vi "GBF Face avant.vi"() -> ()   [LabVIEW 2024]
uses:
  <vilib>/measure/NI_MABase.lvlib
panel:
  in  "reset signal":bool caption="réinitialisation du signal"
  out "Fréquence":dbl
  in  "N° octave":u8(knob) max=9 step=1 scale=0.0..9.0
  in  "Sib":bool
  in  "Sol#":bool
  in  "Fa#":bool
  in  "Mib":bool
  in  "Do#":bool
  in  "SI":bool
  in  "LA":bool
  in  "SOL":bool
  in  "FA":bool
  in  "MI":bool
  in  "RE":bool
  in  "DO":bool
  in  "signal type":T1(ring) caption="type de signal"
  in  "Atténuation":bool
  in  "sampling info":cluster{"Fs":dbl, "#s":dbl}={"Fs"=100000.0, "#s"=100000.0} caption="Echantillonnage" {"Fs" format="%.2p"}
  in  "Bouton Stop":bool
  out "Signal":waveform(dbl)(graph)={"t0"=timestamp(56 s since 1904-01-01), "dt"=1e-05, "Y"=array[100000 elements]}
  in  "Rapport cyclique (%)":dbl(slide) min=0.0 max=100.0 step=5.0 scale=0.0..100.0
  in  "Amplitude":dbl(knob) min=0.0 max=1.0 step=0.01 scale=0.0..1.0
  # "GENERATEUR 1 OCTAVE"
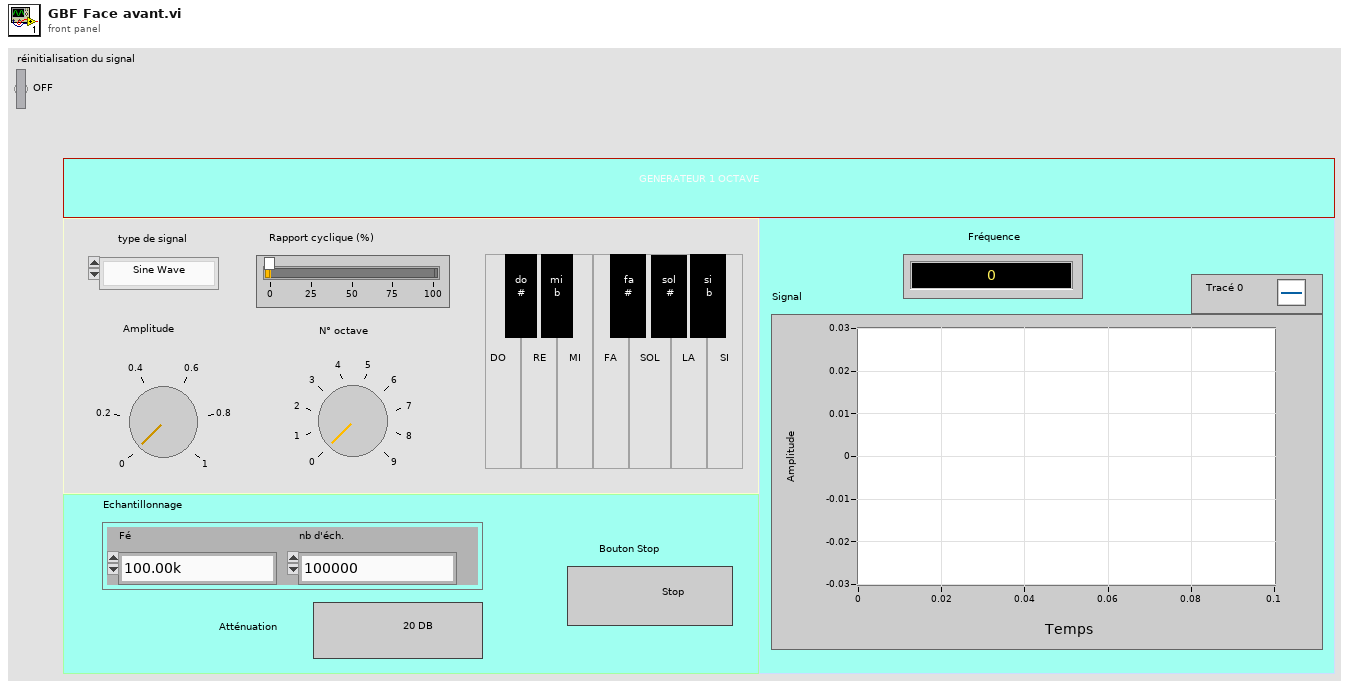
[diagram p1: front panel]
types:
  T1 = enum16{"Sine Wave", "Triangle Wave", "Square Wave", "Sawtooth Wave"}
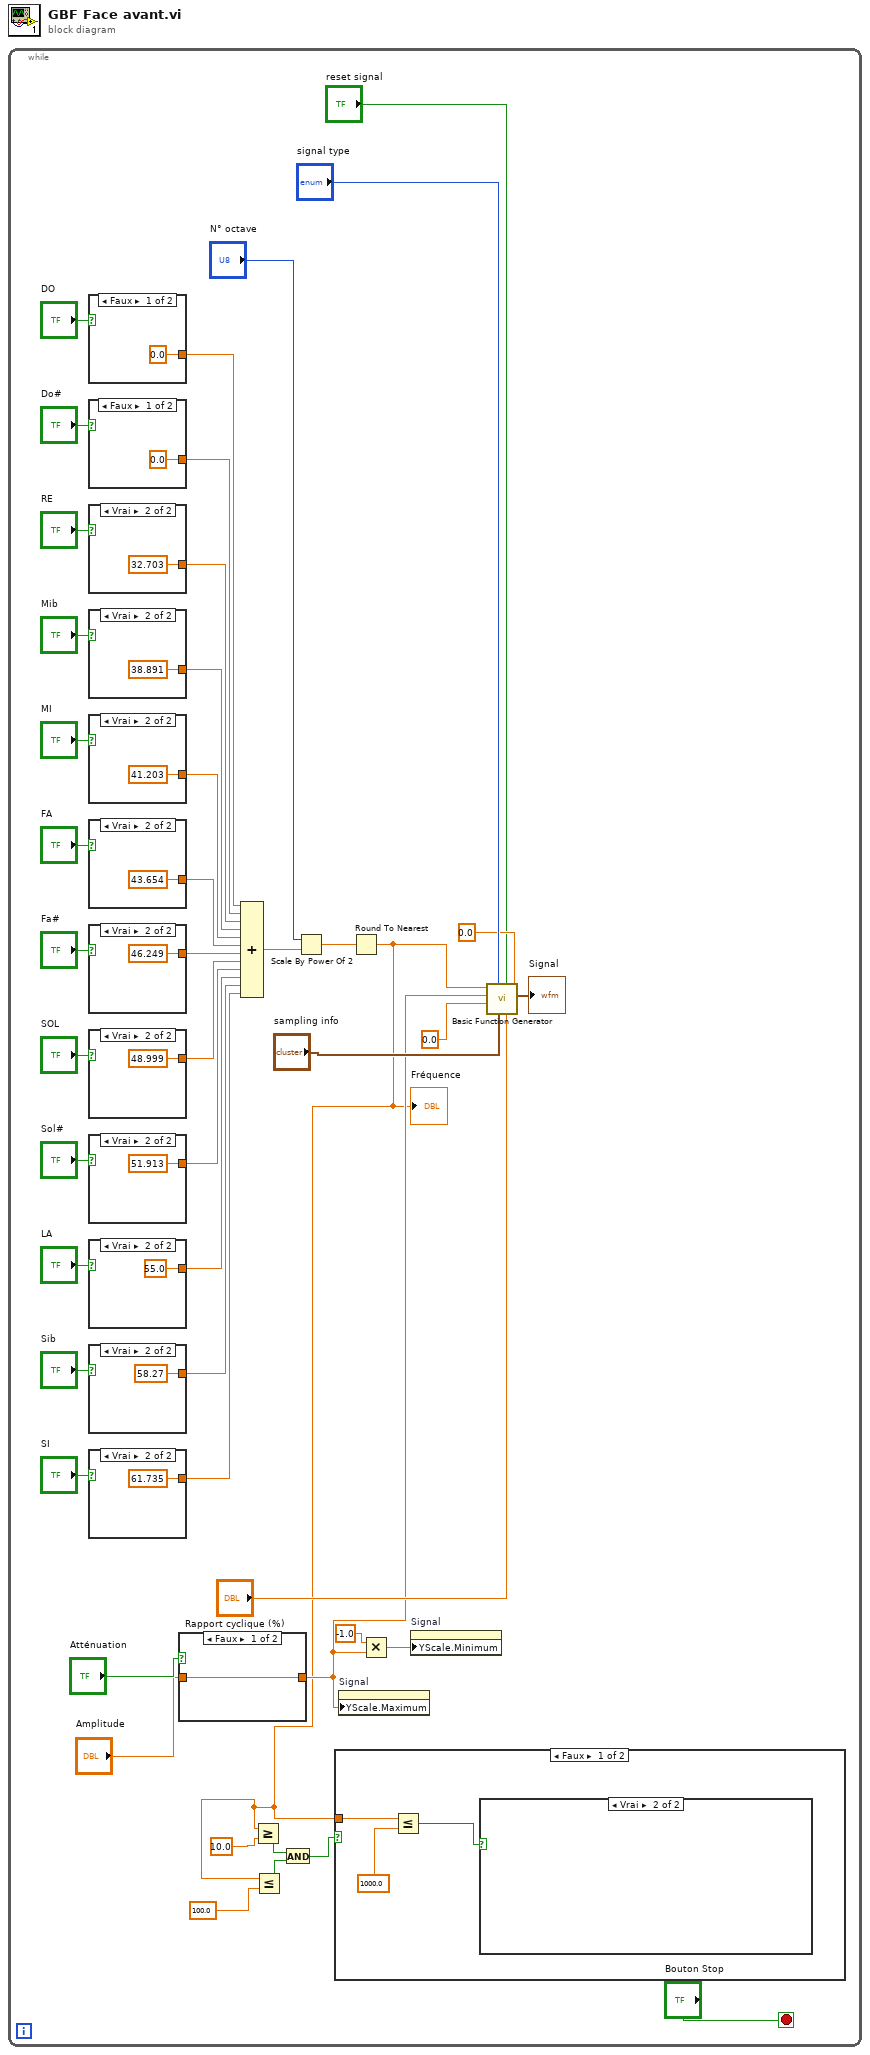
[diagram p0: block diagram]
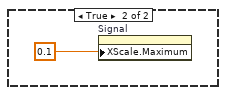
[diagram p3: hidden frame]
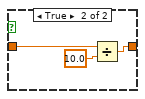
[diagram p4: hidden frame]
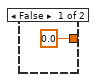
[diagram p5: hidden frame]
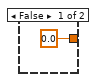
[diagram p6: hidden frame]
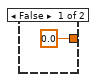
[diagram p7: hidden frame]
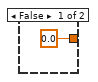
[diagram p8: hidden frame]
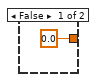
[diagram p9: hidden frame]
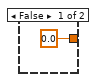
[diagram p10: hidden frame]
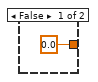
[diagram p11: hidden frame]
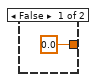
[diagram p12: hidden frame]
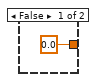
[diagram p13: hidden frame]
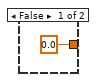
[diagram p14: hidden frame]
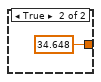
[diagram p15: hidden frame]
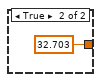
[diagram p16: hidden frame]
diagram:
  n1 = while {
    stop <- "Bouton Stop" stop-if-true
    n2 = case shown="Faux" "DO" {
      tunnel: [0.0 32.703] -> w28
      frame False {
      }
      frame True {
      }
    }
    n3 = case shown="Faux" "Do#" {
      tunnel: [0.0 34.648] -> w27
      frame False {
      }
      frame True {
      }
    }
    n4 = case shown="Vrai" "RE" {
      tunnel: [0.0 32.703] -> w26
      frame False {
      }
      frame True {
      }
    }
    n5 = case shown="Vrai" "Mib" {
      tunnel: [0.0 38.891] -> w25
      frame False {
      }
      frame True {
      }
    }
    n6 = case shown="Vrai" "MI" {
      tunnel: [0.0 41.203] -> w24
      frame False {
      }
      frame True {
      }
    }
    n7 = case shown="Vrai" "FA" {
      tunnel: [0.0 43.654] -> w23
      frame False {
      }
      frame True {
      }
    }
    n8 = case shown="Vrai" "Fa#" {
      tunnel: [0.0 46.249] -> w22
      frame False {
      }
      frame True {
      }
    }
    n9 = case shown="Vrai" "SOL" {
      tunnel: [0.0 48.999] -> w21
      frame False {
      }
      frame True {
      }
    }
    n10 = case shown="Vrai" "Sol#" {
      tunnel: [0.0 51.913] -> w20
      frame False {
      }
      frame True {
      }
    }
    n11 = case shown="Vrai" "LA" {
      tunnel: [0.0 55.0] -> w19
      frame False {
      }
      frame True {
      }
    }
    n12 = case shown="Vrai" "Sib" {
      tunnel: [0.0 58.27] -> w18
      frame False {
      }
      frame True {
      }
    }
    n13 = case shown="Vrai" "SI" {
      tunnel: [0.0 61.735] -> w17
      frame False {
      }
      frame True {
      }
    }
    n14 = case shown="Faux" "Atténuation" {
      tunnel: [w51 w54] -> w8
      tunnel: "Amplitude" -> [w51 w53]
      frame False {
      }
      frame True {
        n15 = Divide(x=w53, y=10.0) -> (x/y=w54:dbl)
      }
    }
    n16 = Compound Arithmetic op=ADD(w28, w27, w26, w25, w24, w23, w22, w21, w20, w19, w18, w17) -> (w16:dbl)
    n17 = Scale By Power Of 2(n="N° octave", x=w16) -> (x*2^n=w10:dbl)
    n18 = property on="Signal" class="GraphWF (strict)"("YScale.Maximum"=w8) -> ()  [unwired: 2 in, 2 out]
    n19 = Round To Nearest(number=w10) -> (nearest integer value=w1:dbl)
    "Fréquence" <- w1
    n20 = Greater Or Equal?(x=w1, y=10.0) -> (x >= y?=w4:bool)
    n21 = Less Or Equal?(x=w1, y=100.0) -> (x <= y?=w3:bool)
    n22 = And(x=w4, y=w3) -> (x .and. y?=w2:bool)
    n23 = case shown="Faux" w2 {
      tunnel: w1 -> [w48 _]
      frame False {
        n24 = Less Or Equal?(x=w48, y=1000.0) -> (x <= y?=w49:bool)
        n25 = case shown="Vrai" w49 {
          frame False {
          }
          frame True {
          }
        }
      }
      frame True {
        n26 = property on="Signal" class="GraphWF (strict)"("XScale.Maximum"=0.1) -> ()  [unwired: 2 in, 2 out]
      }
    }
    n27 = Multiply(x=-1.0, y=w8) -> (x*y=w7:dbl)
    n28 = property on="Signal" class="GraphWF (strict)"("YScale.Minimum"=w7) -> ()  [unwired: 2 in, 2 out]
    n29 = call <vilib>:"Basic Function Generator.vi"("offset"=0.0, "square wave duty cycle (%)"="Rapport cyclique (%)", "reset signal"="reset signal", "sampling info"="sampling info", "signal type"="signal type", "phase"=0.0, "amplitude"=w8, "frequency"=w1) -> ("signal out"=→"Signal":waveform(dbl))  [unwired: 1 in, 2 out]
  }
